vi "TDC_getChainPosition.vi"(8 "Error In":errorcluster) -> (0 "Error Out":errorcluster, 1 "Length":i32, 2 "Position":i32)   [LabVIEW 2011]
uses:
  tdcbase.dll
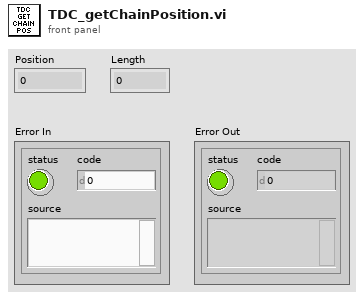
[diagram p1: front panel]
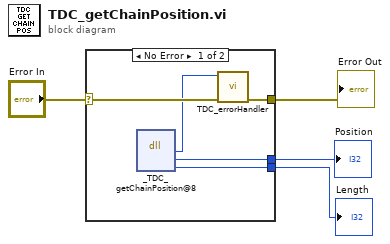
[diagram p0: block diagram]
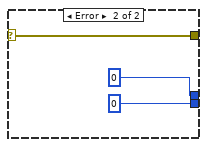
[diagram p2: hidden frame]
diagram:
  n1 = case shown="No Error" "Error In" {
    selector: "Error In" -> [w8 w12]
    tunnel: [w7 w12] -> w3
    tunnel: [w9 0] -> w1
    tunnel: [w5 0] -> w2
    frame No Error {
      n2 = dll-call lib="X:/tdcbase.dll" fn="_TDC_getChainPosition@8"() -> ("return type"=w6:i32, "position"=w9:i32, "length"=w5:i32)  [unwired: 5 in, 2 out]
      n3 = call "TDC_errorHandler.vi"("Error In"=w8, "TDC Return Code"=w6) -> ("Error Out"=w7:errorcluster)  [unwired: 9 in]
    }
    frame Error {
    }
  }
  "Error Out" <- w3
  "Position" <- w1
  "Length" <- w2
